vi "Read Manifold Parameters.vi"(8 "error in":errorcluster, 11 "Config Manager in":refnum<class "Config Manager Class.lvclass">) -> (0 "error out":errorcluster, 1 "Ports":T1[](array[typedef]), 2 "Channels":T2[](array[typedef]), 3 "Config Manager out":refnum<class "Config Manager Class.lvclass">)   [LabVIEW 2017, in "Config Manager Class.lvclass"]
uses:
  Config Manager Class.lvclass
  WorkTable Class/Type Definitions/Worktable_Manifold Channel Names.ctl
  WorkTable Class/Type Definitions/Worktable_Manifold Channel.ctl
  Config Manager Class.lvclass/Config Manager Class.ctl
  <vilib>/Utility/config.llb/Read Key (String).vi
  <vilib>/Utility/config.llb/NI_LVConfig.lvlib
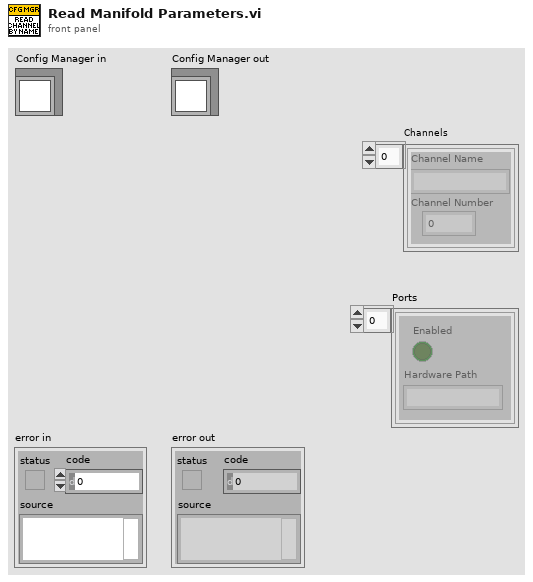
[diagram p1: front panel]
types:
  T1 = typedef "Worktable_Manifold Channel.ctl" = cluster{"Enabled":bool, "Hardware Path":string}
  T2 = typedef "Worktable_Manifold Channel Names.ctl" = cluster{"Channel Name":string, "Channel Number":i8}
  T3 = typedef "NI_LVConfig.lvlib/Config Data RefNum.ctl" = refnum<k1>
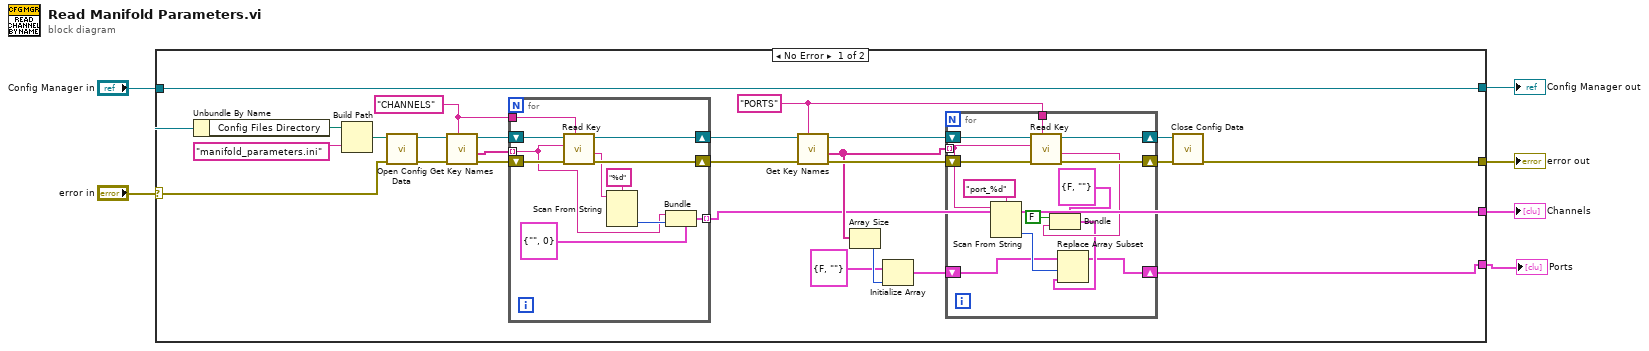
[diagram p0: block diagram]
diagram:
  n1 = case shown="No Error" "error in" {
    selector: "error in" -> [w31 w58]
    tunnel: [w29 w58] -> w4
    tunnel: [w22 w57] -> w3
    tunnel: "Config Manager in" -> [w22 w57]
    tunnel: [w8 _] -> w2
    tunnel: [w7 _] -> w1
    frame No Error {
      w17 = "PORTS" ("section")
      w16 = "CHANNELS" ("section")
      n2 = Unbundle By Name(w22) -> ("Config Files Directory"=w21:path)
      n3 = Build Path(base path=w21, name or relative path="manifold_parameters.ini") -> (appended path=w28:path)
      n4 = call <vilib>:"Open Config Data.vi"("error in (no error)"=w31, "configuration file path"=w28) -> ("error out"=w25:errorcluster, "refnum"=w24:T3)  [unwired: 7 in, 1 out]
      n5 = call <vilib>:"Get Key Names.vi"("section"=w16, "error in (no error)"=w25, "refnum"=w24) -> ("error out"=w26:errorcluster, "key names"=w15:string[], "refnum out"=w27:T3)  [unwired: 5 in, 1 out]
      n6 = for {
        shift-right: [w54] -> w20
        shift-left: w27 -> [w56]
        shift-right: [w53] -> w18
        shift-left: w26 -> [w55]
        tunnel: w16 -> [w52]
        tunnel: w15 -> [w47] mode=indexing
        tunnel: [w46] -> w8 mode=indexing
        n7 = call-poly <vilib>:"Read Key.vi"("section"=w52, "error in (no error)"=w55, "key"=w47, "refnum"=w56) -> ("error out"=w53:errorcluster, "value"=w49:string, "refnum out"=w54:T3)  [unwired: 4 in, 1 out]
        n8 = Scan From String(format string="%d", input string=w49) -> (output 1=w50:i32)  [unwired: 3 in, 3 out]
        n9 = Bundle(cluster=T2 {"Channel Name"="", "Channel Number"=0} ("Vacuum Channel Names"), "Channel Name"=w47, "Channel Number"=w50) -> (w46:T2)
      }
      n10 = call <vilib>:"Get Key Names.vi"("section"=w17, "error in (no error)"=w18, "refnum"=w20) -> ("error out"=w14:errorcluster, "key names"=w13:string[], "refnum out"=w19:T3)  [unwired: 5 in, 1 out]
      n11 = Array Size(array=w13) -> (size(s)=w12:i32)
      n12 = Initialize Array(T1 {"Enabled"=FALSE, "Hardware Path"=""} ("Vacuum Channel Status"), w12) -> (w10:T1[])
      n13 = for {
        tunnel: w17 -> [w43]
        shift-right: [w45] -> w23
        shift-left: w19 -> [w44]
        shift-right: [w41] -> w9
        shift-left: w14 -> [w42]
        tunnel: w13 -> [w39] mode=indexing
        shift-right: [w33] -> w7
        shift-left: w10 -> [w37]
        n14 = Scan From String(format string="port_%d", input string=w39) -> (output 1=w38:i32)  [unwired: 3 in, 3 out]
        n15 = call-poly <vilib>:"Read Key.vi"("section"=w43, "error in (no error)"=w42, "key"=w39, "refnum"=w44) -> ("error out"=w41:errorcluster, "value"=w35:string, "refnum out"=w45:T3)  [unwired: 4 in, 1 out]
        n16 = Bundle(cluster=T1 {"Enabled"=FALSE, "Hardware Path"=""} ("Vacuum Channel Status"), "Enabled"=FALSE, "Hardware Path"=w35) -> (w34:T1)
        n17 = Replace Array Subset(array=w37, new element=w34, index=w38) -> (w33:T1[])
      }
      n18 = call <vilib>:"Close Config Data.vi"("error in (no error)"=w9, "refnum"=w23) -> ("error out"=w29:errorcluster)  [unwired: 8 in, 1 out]
    }
    frame Error {
    }
  }
  "error out" <- w4
  "Config Manager out" <- w3
  "Ports" <- w1
  "Channels" <- w2
